vi "InGaAs-GaAs QDSL-111222b- diff GIT - same T.vi"() -> ()   [LabVIEW 2011]
panel:
  out "step number  5":i32
  in  "Number of \nGrowth Steps 5":i32=10
  out "step number  4":i32
  in  "Number of \nGrowth Steps 4":i32=10
  out "step number  3":i32
  in  "Number of \nGrowth Steps 3":i32=10
  out "step number  2":i32
  in  "Number of \nGrowth Steps 2":i32=10
  in  "Indium Flow 2":dbl=37.6
  in  "Ga Flow 3":dbl=4.2
  in  "Ga Flow 2":dbl=4.2
  in  "Ga Flow 1":dbl=4.2
  in  "Indium Flow":dbl=37.6
  in  "Number of \nGrowth Steps":i32=10
  out "step number":i32
  in  "As_Gas Flow":dbl=3.5
  in  "Manifold H2 Flow":dbl=720.0
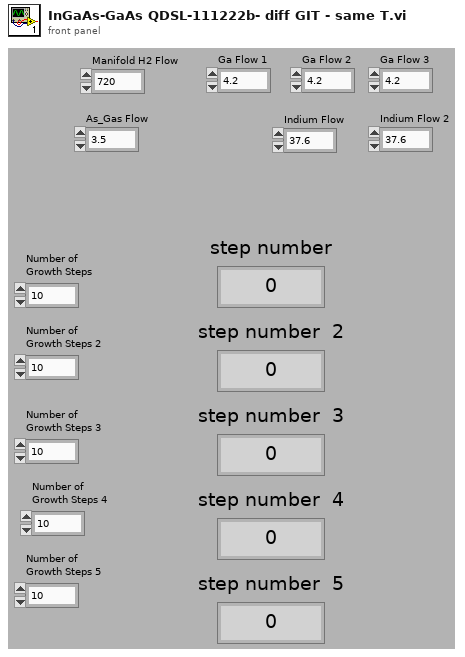
[diagram p1: front panel]
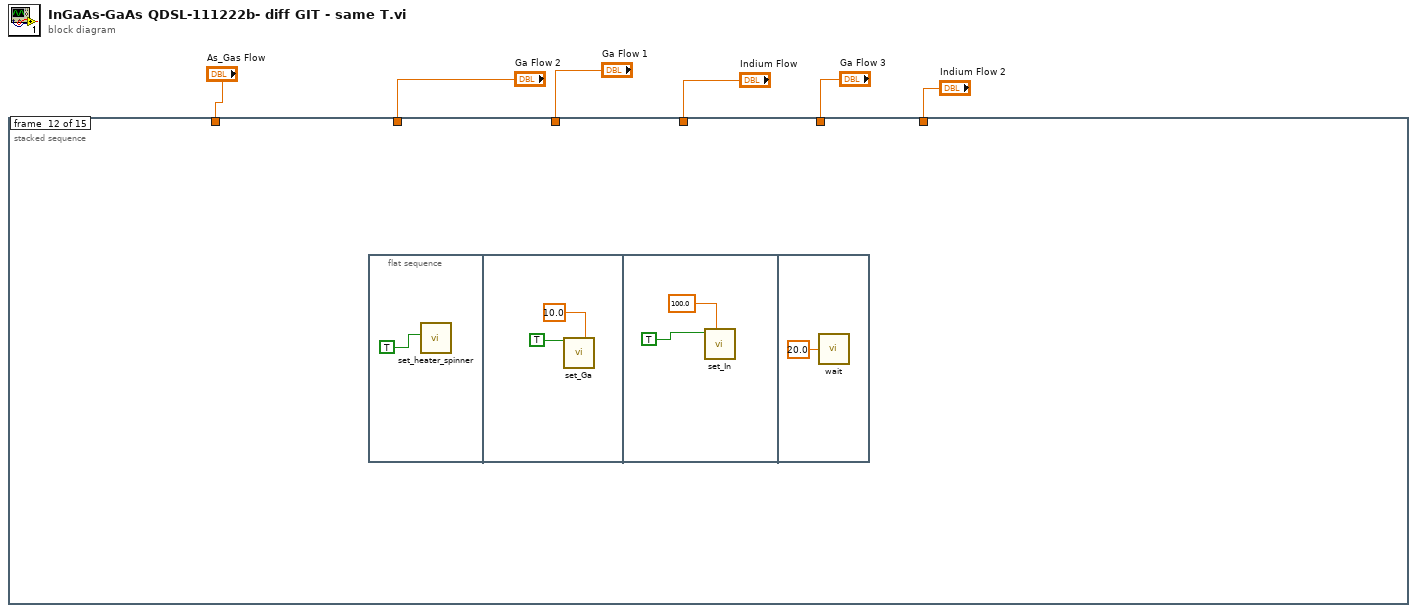
[diagram p0: block diagram]
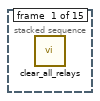
[diagram p2: hidden frame]
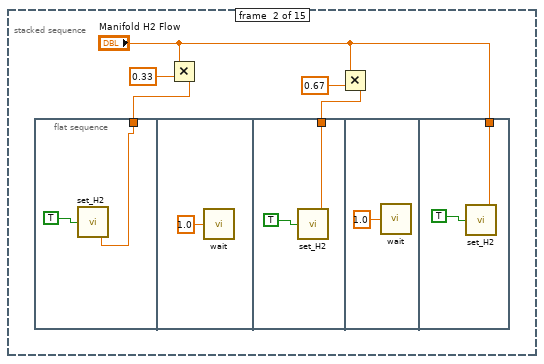
[diagram p3: hidden frame]
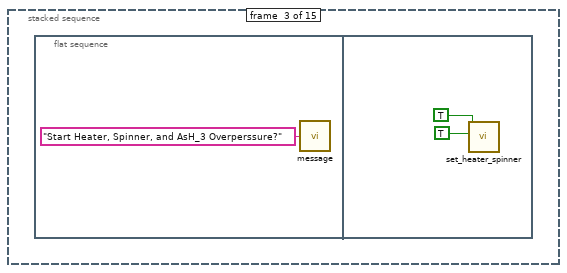
[diagram p4: hidden frame]
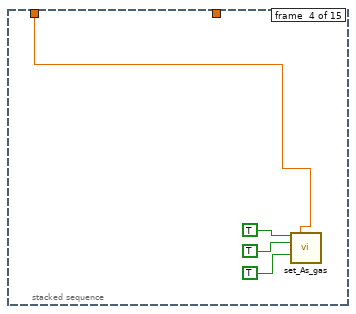
[diagram p5: hidden frame]
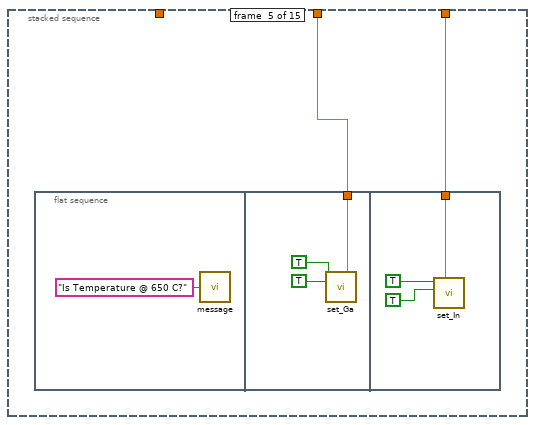
[diagram p6: hidden frame]
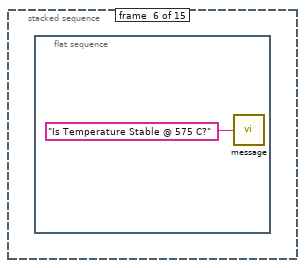
[diagram p7: hidden frame]
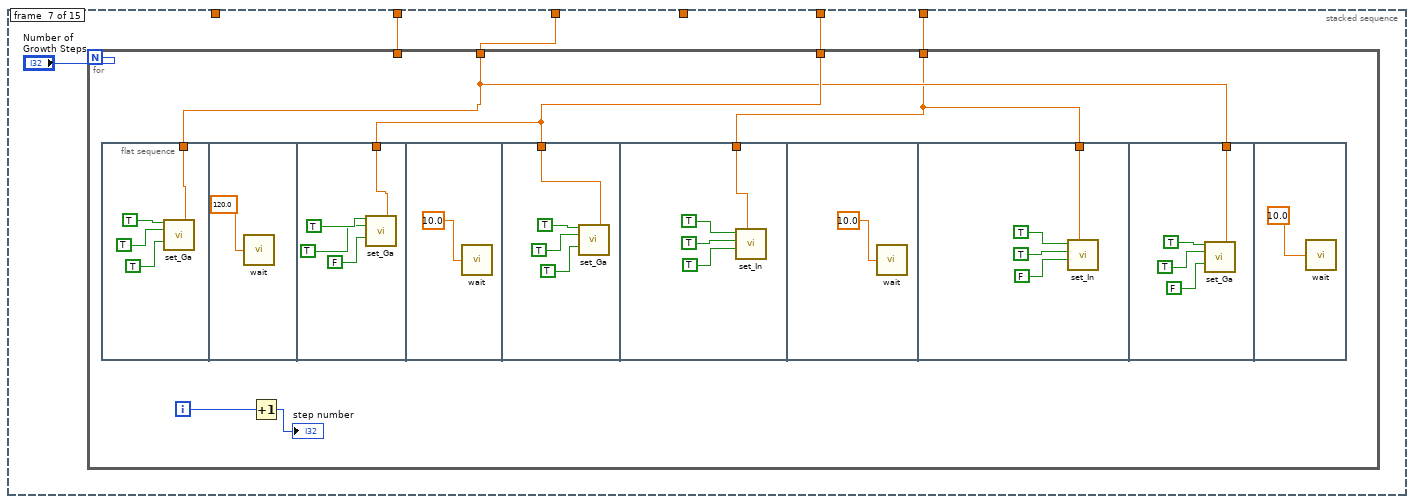
[diagram p8: hidden frame]
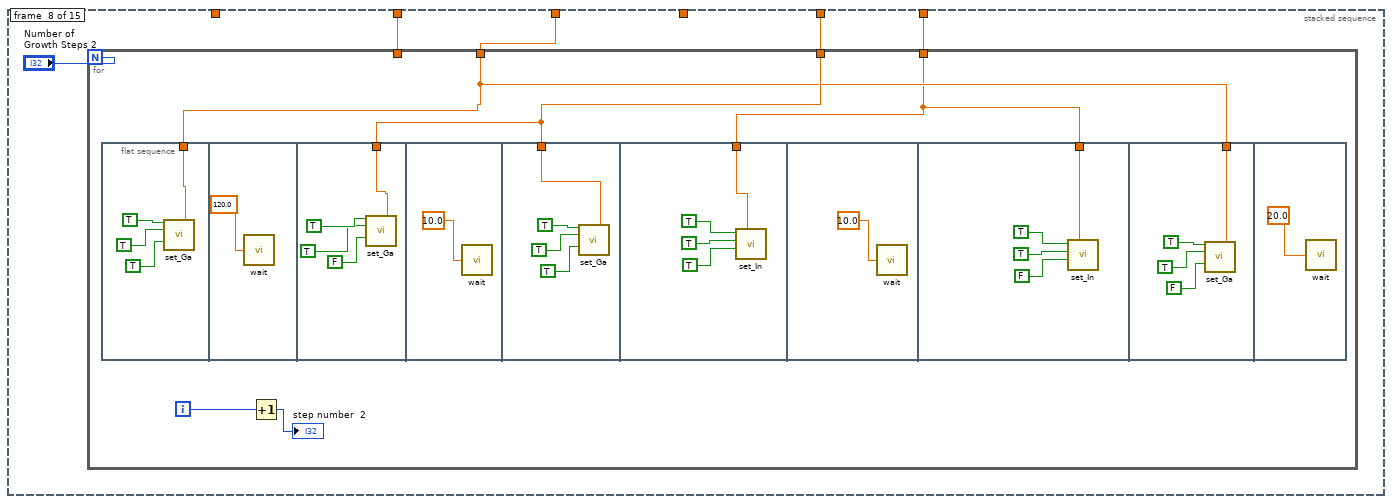
[diagram p9: hidden frame]
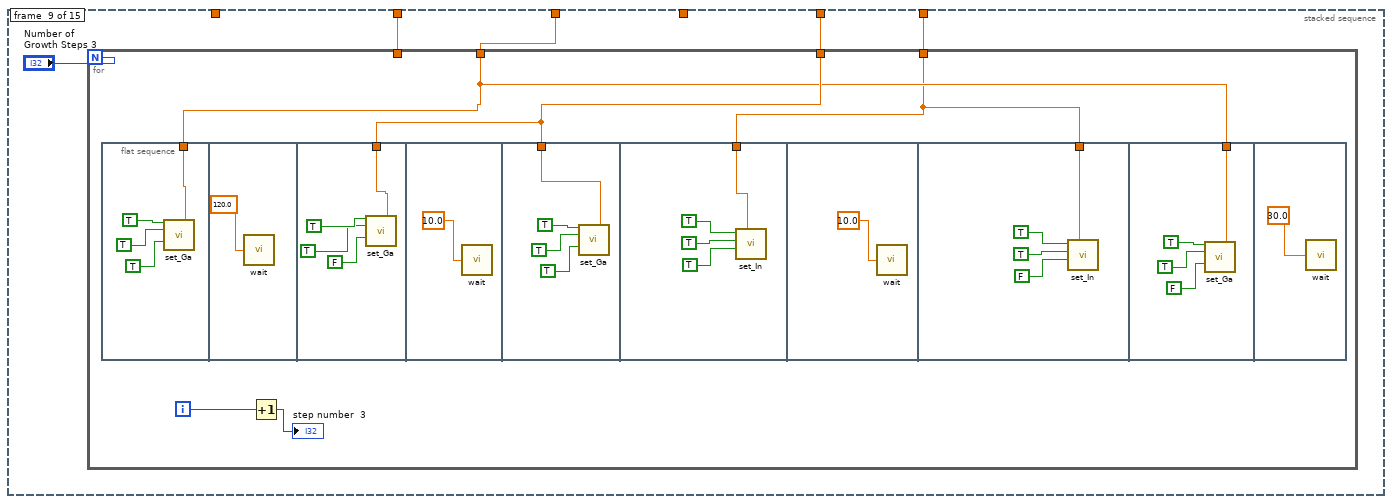
[diagram p10: hidden frame]
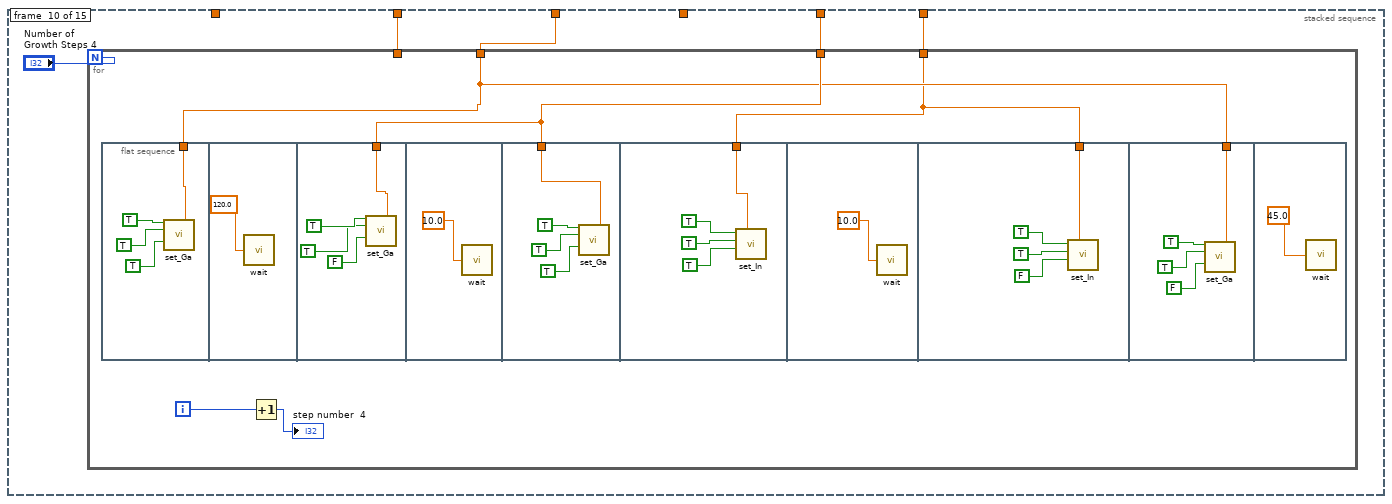
[diagram p11: hidden frame]
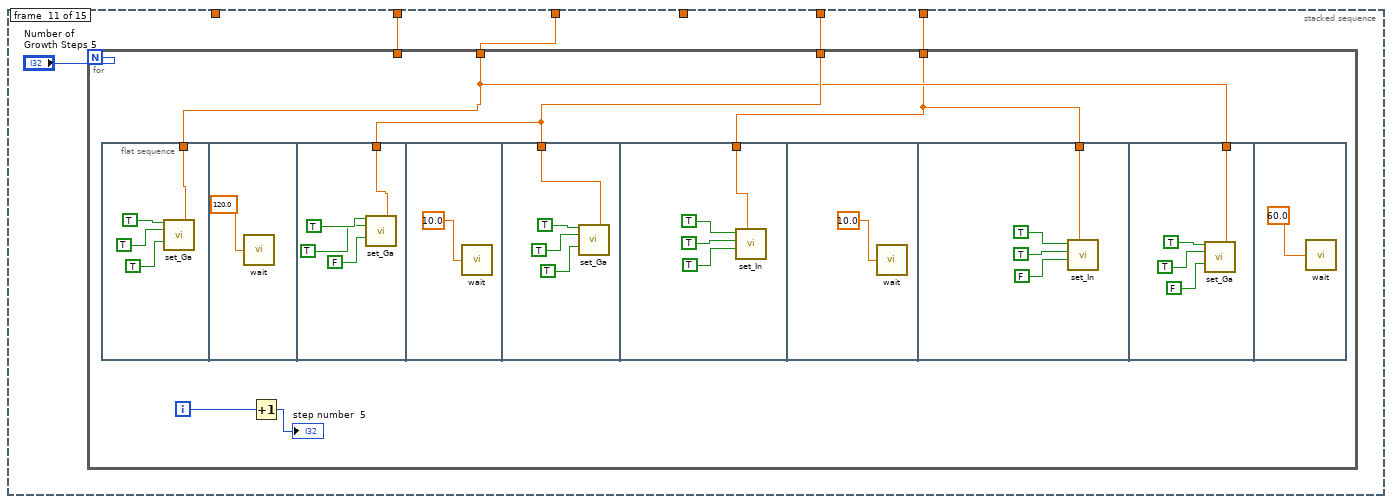
[diagram p12: hidden frame]
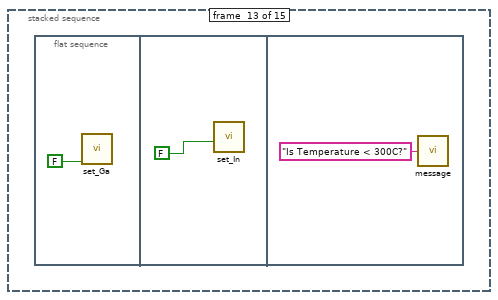
[diagram p13: hidden frame]
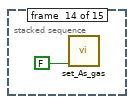
[diagram p14: hidden frame]
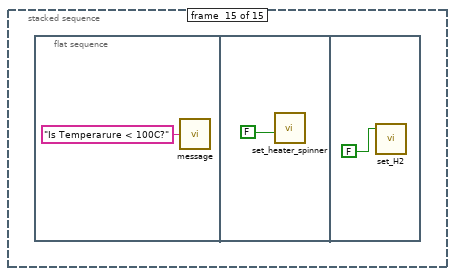
[diagram p15: hidden frame]
diagram:
  n1 = stacked-sequence {
    tunnel: "Ga Flow 1" -> [_ _ _ _ w28 _ w40 w78 w116 w154 w192 _ _ _ _]
    tunnel: "As_Gas Flow" -> [_ _ _ w23 _ _ _ _ _ _ _ _ _ _ _]
    tunnel: "Indium Flow" -> [_ _ _ _ w27 _ _ _ _ _ _ _ _ _ _]
    tunnel: "Ga Flow 2" -> [_ _ _ _ _ _ w39 w77 w115 w153 w191 _ _ _ _]
    tunnel: "Ga Flow 3" -> [_ _ _ _ _ _ w38 w76 w114 w152 w190 _ _ _ _]
    tunnel: "Indium Flow 2" -> [_ _ _ _ _ _ w37 w75 w113 w151 w189 _ _ _ _]
    frame #0 {
      n2 = call "clear_all_relays.vi"() -> ()  [unwired: 2 out]
    }
    frame #1 {
      n3 = flat-sequence {
        tunnel: w11 -> [w12]
        tunnel: w9 -> [w15]
        tunnel: "Manifold H2 Flow" -> [w18]
        frame #0 {
          n4 = call "set_H2.vi"("Manifold H2 Flow"=w12, "H2 Active"=TRUE) -> ()  [unwired: 2 in, 2 out]
        }
        frame #1 {
          n5 = call "wait.vi"("Wait (s)"=1.0) -> ()
        }
        frame #2 {
          n6 = call "set_H2.vi"("Manifold H2 Flow"=w15, "H2 Active"=TRUE) -> ()  [unwired: 2 in, 2 out]
        }
        frame #3 {
          n7 = call "wait.vi"("Wait (s)"=1.0) -> ()
        }
        frame #4 {
          n8 = call "set_H2.vi"("Manifold H2 Flow"=w18, "H2 Active"=TRUE) -> ()  [unwired: 2 in, 2 out]
        }
      }
      n9 = Multiply(x="Manifold H2 Flow", y=0.33) -> (x*y=w11:dbl)
      n10 = Multiply(x="Manifold H2 Flow", y=0.67) -> (x*y=w9:dbl)
    }
    frame #2 {
      n11 = flat-sequence {
        frame #0 {
          n12 = call "message.vi"("message"="Start Heater, Spinner, and AsH_3 Overperssure?") -> ()
        }
        frame #1 {
          n13 = call "set_heater_spinner.vi"("Spinner"=TRUE, "Heater"=TRUE) -> ()  [unwired: 1 in, 7 out]
        }
      }
    }
    frame #3 {
      n14 = call "set_As_gas.vi"("As_Gas Active"=TRUE, "As_Gas Flow"=w23, "As_Gas In"=TRUE, "As_Gas Run"=TRUE) -> ()  [unwired: 2 in, 10 out]
    }
    frame #4 {
      n15 = flat-sequence {
        tunnel: w28 -> [w30]
        tunnel: w27 -> [w33]
        frame #0 {
          n16 = call "message.vi"("message"="Is Temperature @ 650 C?") -> ()
        }
        frame #1 {
          n17 = call "set_Ga.vi"("Ga Active"=TRUE, "Ga Flow 1"=w30, "Ga Bubbler"=TRUE) -> ()  [unwired: 5 in, 8 out]
        }
        frame #2 {
          n18 = call "set_In.vi"("Indium Flow"=w33, "In Bubbler"=TRUE ("Ga Bubbler"), "In Active"=TRUE ("Ga Active")) -> ()  [unwired: 2 in, 5 out]
        }
      }
    }
    frame #5 {
      n19 = flat-sequence {
        frame #0 {
          n20 = call "message.vi"("message"="Is Temperature Stable @ 575 C?") -> ()
        }
      }
    }
    frame #6 {
      n21 = for {
        N: "Number of \nGrowth Steps" -> [_]
        tunnel: w40 -> [w43]
        tunnel: w39 -> [_]
        tunnel: w38 -> [w44]
        tunnel: w37 -> [w42]
        i -> [w45]
        n22 = flat-sequence {
          tunnel: w43 -> [w47]
          tunnel: w44 -> [w52]
          tunnel: w44 -> [w57]
          tunnel: w42 -> [w61]
          tunnel: w42 -> [w66]
          tunnel: w43 -> [w70]
          frame #0 {
            n23 = call "set_Ga.vi"("Ga Active"=TRUE ("P_Gas Active"), "Ga Flow 1"=w47, "Ga Bubbler"=TRUE ("P_Gas In"), "Ga Run"=TRUE ("P_Gas Run")) -> ()  [unwired: 4 in, 8 out]
          }
          frame #1 {
            n24 = call "wait.vi"("Wait (s)"=120.0) -> ()
          }
          frame #2 {
            n25 = call "set_Ga.vi"("Ga Active"=TRUE ("P_Gas Active"), "Ga Flow 1"=w52, "Ga Bubbler"=TRUE ("P_Gas In"), "Ga Run"=FALSE ("P_Gas Run")) -> ()  [unwired: 4 in, 8 out]
          }
          frame #3 {
            n26 = call "wait.vi"("Wait (s)"=10.0) -> ()
          }
          frame #4 {
            n27 = call "set_Ga.vi"("Ga Active"=TRUE ("P_Gas Active"), "Ga Flow 1"=w57, "Ga Bubbler"=TRUE ("P_Gas In"), "Ga Run"=TRUE ("P_Gas Run")) -> ()  [unwired: 4 in, 8 out]
          }
          frame #5 {
            n28 = call "set_In.vi"("Indium Flow"=w61, "In Run"=TRUE ("P_Gas Run"), "In Bubbler"=TRUE ("P_Gas In"), "In Active"=TRUE ("P_Gas Active")) -> ()  [unwired: 1 in, 5 out]
          }
          frame #6 {
            n29 = call "wait.vi"("Wait (s)"=10.0) -> ()
          }
          frame #7 {
            n30 = call "set_In.vi"("Indium Flow"=w66, "In Run"=FALSE ("P_Gas Run"), "In Bubbler"=TRUE ("P_Gas In"), "In Active"=TRUE ("P_Gas Active")) -> ()  [unwired: 1 in, 5 out]
          }
          frame #8 {
            n31 = call "set_Ga.vi"("Ga Active"=TRUE ("P_Gas Active"), "Ga Flow 1"=w70, "Ga Bubbler"=TRUE ("P_Gas In"), "Ga Run"=FALSE ("P_Gas Run")) -> ()  [unwired: 4 in, 8 out]
          }
          frame #9 {
            n32 = call "wait.vi"("Wait (s)"=10.0) -> ()
          }
        }
        n33 = Increment(x=w45) -> (x+1=→"step number":i32)
      }
    }
    frame #7 {
      n34 = for {
        N: "Number of \nGrowth Steps 2" -> [_]
        tunnel: w78 -> [w81]
        tunnel: w77 -> [_]
        tunnel: w76 -> [w82]
        tunnel: w75 -> [w80]
        i -> [w83]
        n35 = flat-sequence {
          tunnel: w81 -> [w85]
          tunnel: w82 -> [w90]
          tunnel: w82 -> [w95]
          tunnel: w80 -> [w99]
          tunnel: w80 -> [w104]
          tunnel: w81 -> [w108]
          frame #0 {
            n36 = call "set_Ga.vi"("Ga Active"=TRUE ("P_Gas Active"), "Ga Flow 1"=w85, "Ga Bubbler"=TRUE ("P_Gas In"), "Ga Run"=TRUE ("P_Gas Run")) -> ()  [unwired: 4 in, 8 out]
          }
          frame #1 {
            n37 = call "wait.vi"("Wait (s)"=120.0) -> ()
          }
          frame #2 {
            n38 = call "set_Ga.vi"("Ga Active"=TRUE ("P_Gas Active"), "Ga Flow 1"=w90, "Ga Bubbler"=TRUE ("P_Gas In"), "Ga Run"=FALSE ("P_Gas Run")) -> ()  [unwired: 4 in, 8 out]
          }
          frame #3 {
            n39 = call "wait.vi"("Wait (s)"=10.0) -> ()
          }
          frame #4 {
            n40 = call "set_Ga.vi"("Ga Active"=TRUE ("P_Gas Active"), "Ga Flow 1"=w95, "Ga Bubbler"=TRUE ("P_Gas In"), "Ga Run"=TRUE ("P_Gas Run")) -> ()  [unwired: 4 in, 8 out]
          }
          frame #5 {
            n41 = call "set_In.vi"("Indium Flow"=w99, "In Run"=TRUE ("P_Gas Run"), "In Bubbler"=TRUE ("P_Gas In"), "In Active"=TRUE ("P_Gas Active")) -> ()  [unwired: 1 in, 5 out]
          }
          frame #6 {
            n42 = call "wait.vi"("Wait (s)"=10.0) -> ()
          }
          frame #7 {
            n43 = call "set_In.vi"("Indium Flow"=w104, "In Run"=FALSE ("P_Gas Run"), "In Bubbler"=TRUE ("P_Gas In"), "In Active"=TRUE ("P_Gas Active")) -> ()  [unwired: 1 in, 5 out]
          }
          frame #8 {
            n44 = call "set_Ga.vi"("Ga Active"=TRUE ("P_Gas Active"), "Ga Flow 1"=w108, "Ga Bubbler"=TRUE ("P_Gas In"), "Ga Run"=FALSE ("P_Gas Run")) -> ()  [unwired: 4 in, 8 out]
          }
          frame #9 {
            n45 = call "wait.vi"("Wait (s)"=20.0) -> ()
          }
        }
        n46 = Increment(x=w83) -> (x+1=→"step number  2":i32)
      }
    }
    frame #8 {
      n47 = for {
        N: "Number of \nGrowth Steps 3" -> [_]
        tunnel: w116 -> [w119]
        tunnel: w115 -> [_]
        tunnel: w114 -> [w120]
        tunnel: w113 -> [w118]
        i -> [w121]
        n48 = flat-sequence {
          tunnel: w119 -> [w123]
          tunnel: w120 -> [w128]
          tunnel: w120 -> [w133]
          tunnel: w118 -> [w137]
          tunnel: w118 -> [w142]
          tunnel: w119 -> [w146]
          frame #0 {
            n49 = call "set_Ga.vi"("Ga Active"=TRUE ("P_Gas Active"), "Ga Flow 1"=w123, "Ga Bubbler"=TRUE ("P_Gas In"), "Ga Run"=TRUE ("P_Gas Run")) -> ()  [unwired: 4 in, 8 out]
          }
          frame #1 {
            n50 = call "wait.vi"("Wait (s)"=120.0) -> ()
          }
          frame #2 {
            n51 = call "set_Ga.vi"("Ga Active"=TRUE ("P_Gas Active"), "Ga Flow 1"=w128, "Ga Bubbler"=TRUE ("P_Gas In"), "Ga Run"=FALSE ("P_Gas Run")) -> ()  [unwired: 4 in, 8 out]
          }
          frame #3 {
            n52 = call "wait.vi"("Wait (s)"=10.0) -> ()
          }
          frame #4 {
            n53 = call "set_Ga.vi"("Ga Active"=TRUE ("P_Gas Active"), "Ga Flow 1"=w133, "Ga Bubbler"=TRUE ("P_Gas In"), "Ga Run"=TRUE ("P_Gas Run")) -> ()  [unwired: 4 in, 8 out]
          }
          frame #5 {
            n54 = call "set_In.vi"("Indium Flow"=w137, "In Run"=TRUE ("P_Gas Run"), "In Bubbler"=TRUE ("P_Gas In"), "In Active"=TRUE ("P_Gas Active")) -> ()  [unwired: 1 in, 5 out]
          }
          frame #6 {
            n55 = call "wait.vi"("Wait (s)"=10.0) -> ()
          }
          frame #7 {
            n56 = call "set_In.vi"("Indium Flow"=w142, "In Run"=FALSE ("P_Gas Run"), "In Bubbler"=TRUE ("P_Gas In"), "In Active"=TRUE ("P_Gas Active")) -> ()  [unwired: 1 in, 5 out]
          }
          frame #8 {
            n57 = call "set_Ga.vi"("Ga Active"=TRUE ("P_Gas Active"), "Ga Flow 1"=w146, "Ga Bubbler"=TRUE ("P_Gas In"), "Ga Run"=FALSE ("P_Gas Run")) -> ()  [unwired: 4 in, 8 out]
          }
          frame #9 {
            n58 = call "wait.vi"("Wait (s)"=30.0) -> ()
          }
        }
        n59 = Increment(x=w121) -> (x+1=→"step number  3":i32)
      }
    }
    frame #9 {
      n60 = for {
        N: "Number of \nGrowth Steps 4" -> [_]
        tunnel: w154 -> [w157]
        tunnel: w153 -> [_]
        tunnel: w152 -> [w158]
        tunnel: w151 -> [w156]
        i -> [w159]
        n61 = flat-sequence {
          tunnel: w157 -> [w161]
          tunnel: w158 -> [w166]
          tunnel: w158 -> [w171]
          tunnel: w156 -> [w175]
          tunnel: w156 -> [w180]
          tunnel: w157 -> [w184]
          frame #0 {
            n62 = call "set_Ga.vi"("Ga Active"=TRUE ("P_Gas Active"), "Ga Flow 1"=w161, "Ga Bubbler"=TRUE ("P_Gas In"), "Ga Run"=TRUE ("P_Gas Run")) -> ()  [unwired: 4 in, 8 out]
          }
          frame #1 {
            n63 = call "wait.vi"("Wait (s)"=120.0) -> ()
          }
          frame #2 {
            n64 = call "set_Ga.vi"("Ga Active"=TRUE ("P_Gas Active"), "Ga Flow 1"=w166, "Ga Bubbler"=TRUE ("P_Gas In"), "Ga Run"=FALSE ("P_Gas Run")) -> ()  [unwired: 4 in, 8 out]
          }
          frame #3 {
            n65 = call "wait.vi"("Wait (s)"=10.0) -> ()
          }
          frame #4 {
            n66 = call "set_Ga.vi"("Ga Active"=TRUE ("P_Gas Active"), "Ga Flow 1"=w171, "Ga Bubbler"=TRUE ("P_Gas In"), "Ga Run"=TRUE ("P_Gas Run")) -> ()  [unwired: 4 in, 8 out]
          }
          frame #5 {
            n67 = call "set_In.vi"("Indium Flow"=w175, "In Run"=TRUE ("P_Gas Run"), "In Bubbler"=TRUE ("P_Gas In"), "In Active"=TRUE ("P_Gas Active")) -> ()  [unwired: 1 in, 5 out]
          }
          frame #6 {
            n68 = call "wait.vi"("Wait (s)"=10.0) -> ()
          }
          frame #7 {
            n69 = call "set_In.vi"("Indium Flow"=w180, "In Run"=FALSE ("P_Gas Run"), "In Bubbler"=TRUE ("P_Gas In"), "In Active"=TRUE ("P_Gas Active")) -> ()  [unwired: 1 in, 5 out]
          }
          frame #8 {
            n70 = call "set_Ga.vi"("Ga Active"=TRUE ("P_Gas Active"), "Ga Flow 1"=w184, "Ga Bubbler"=TRUE ("P_Gas In"), "Ga Run"=FALSE ("P_Gas Run")) -> ()  [unwired: 4 in, 8 out]
          }
          frame #9 {
            n71 = call "wait.vi"("Wait (s)"=45.0) -> ()
          }
        }
        n72 = Increment(x=w159) -> (x+1=→"step number  4":i32)
      }
    }
    frame #10 {
      n73 = for {
        N: "Number of \nGrowth Steps 5" -> [_]
        tunnel: w192 -> [w195]
        tunnel: w191 -> [_]
        tunnel: w190 -> [w196]
        tunnel: w189 -> [w194]
        i -> [w197]
        n74 = flat-sequence {
          tunnel: w195 -> [w199]
          tunnel: w196 -> [w204]
          tunnel: w196 -> [w209]
          tunnel: w194 -> [w213]
          tunnel: w194 -> [w218]
          tunnel: w195 -> [w222]
          frame #0 {
            n75 = call "set_Ga.vi"("Ga Active"=TRUE ("P_Gas Active"), "Ga Flow 1"=w199, "Ga Bubbler"=TRUE ("P_Gas In"), "Ga Run"=TRUE ("P_Gas Run")) -> ()  [unwired: 4 in, 8 out]
          }
          frame #1 {
            n76 = call "wait.vi"("Wait (s)"=120.0) -> ()
          }
          frame #2 {
            n77 = call "set_Ga.vi"("Ga Active"=TRUE ("P_Gas Active"), "Ga Flow 1"=w204, "Ga Bubbler"=TRUE ("P_Gas In"), "Ga Run"=FALSE ("P_Gas Run")) -> ()  [unwired: 4 in, 8 out]
          }
          frame #3 {
            n78 = call "wait.vi"("Wait (s)"=10.0) -> ()
          }
          frame #4 {
            n79 = call "set_Ga.vi"("Ga Active"=TRUE ("P_Gas Active"), "Ga Flow 1"=w209, "Ga Bubbler"=TRUE ("P_Gas In"), "Ga Run"=TRUE ("P_Gas Run")) -> ()  [unwired: 4 in, 8 out]
          }
          frame #5 {
            n80 = call "set_In.vi"("Indium Flow"=w213, "In Run"=TRUE ("P_Gas Run"), "In Bubbler"=TRUE ("P_Gas In"), "In Active"=TRUE ("P_Gas Active")) -> ()  [unwired: 1 in, 5 out]
          }
          frame #6 {
            n81 = call "wait.vi"("Wait (s)"=10.0) -> ()
          }
          frame #7 {
            n82 = call "set_In.vi"("Indium Flow"=w218, "In Run"=FALSE ("P_Gas Run"), "In Bubbler"=TRUE ("P_Gas In"), "In Active"=TRUE ("P_Gas Active")) -> ()  [unwired: 1 in, 5 out]
          }
          frame #8 {
            n83 = call "set_Ga.vi"("Ga Active"=TRUE ("P_Gas Active"), "Ga Flow 1"=w222, "Ga Bubbler"=TRUE ("P_Gas In"), "Ga Run"=FALSE ("P_Gas Run")) -> ()  [unwired: 4 in, 8 out]
          }
          frame #9 {
            n84 = call "wait.vi"("Wait (s)"=60.0) -> ()
          }
        }
        n85 = Increment(x=w197) -> (x+1=→"step number  5":i32)
      }
    }
    frame #11 {
      n86 = flat-sequence {
        frame #0 {
          n87 = call "set_heater_spinner.vi"("Spinner"=TRUE ("Ga Active")) -> ()  [unwired: 2 in, 7 out]
        }
        frame #1 {
          n88 = call "set_Ga.vi"("Ga Active"=TRUE, "Ga Flow 1"=10.0) -> ()  [unwired: 6 in, 8 out]
        }
        frame #2 {
          n89 = call "set_In.vi"("Indium Flow"=100.0 ("Aluminum Flow"), "In Active"=TRUE ("Ga Active")) -> ()  [unwired: 3 in, 5 out]
        }
        frame #3 {
          n90 = call "wait.vi"("Wait (s)"=20.0) -> ()
        }
      }
    }
    frame #12 {
      n91 = flat-sequence {
        frame #0 {
          n92 = call "set_Ga.vi"("Ga Remote"=FALSE) -> ()  [unwired: 7 in, 8 out]
        }
        frame #1 {
          n93 = call "set_In.vi"("In Run"=FALSE ("Ga Remote")) -> ()  [unwired: 4 in, 5 out]
        }
        frame #2 {
          n94 = call "message.vi"("message"="Is Temperature < 300C?") -> ()
        }
      }
    }
    frame #13 {
      n95 = call "set_As_gas.vi"("As_Gas Remote"=FALSE) -> ()  [unwired: 5 in, 10 out]
    }
    frame #14 {
      n96 = flat-sequence {
        frame #0 {
          n97 = call "message.vi"("message"="Is Temperarure < 100C?") -> ()
        }
        frame #1 {
          n98 = call "set_heater_spinner.vi"("Heater/Spinner Remote"=FALSE) -> ()  [unwired: 2 in, 7 out]
        }
        frame #2 {
          n99 = call "set_H2.vi"("H2N2 Remote"=FALSE) -> ()  [unwired: 3 in, 2 out]
        }
      }
    }
  }
